vi "ReedSwitchDistanceGlobal (1).vi"() -> ()   [LabVIEW 2017]
panel:
  in  "Wheel Circumference":dbl=0.835
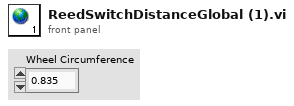
[diagram p1: front panel]
diagram:
